vi "AIT 664 - Write FIFOs.vi"(0 "RT Data in":T2 {"End System Handle" format="%x"; "Label Transfer Config"."Block Data Refs"."Data Reference" format="%.0x"; "Status Config"."Hardware Out Dur Reference" format="%.0x"; "Status Config"."Hardware In Dur Reference" format="%.0x"; "Status Config"."Hardware Out Count Reference" format="%.0x"; "Status Config"."Hardware In Count Reference" format="%.0x"; "Status Config"."Error Data Reference" format="%.0x"; "Hardware Output Tx Channels"."Message Settings"."Transmit Channel Data Reference" format="%.0x"; "Hardware Output Tx Channels"."Message Settings"."Queue Transmit Channel" format="%.0x"; "Hardware Output Tx Channels"."Message Settings"."Driver Data"."Num Bits" min=1 max=32; "Hardware Output Tx Channels"."Message Settings"."Block Data Refs"."Data Reference" format="%.0x"; "Hardware Output Tx Channels"."Rx Com Udp Port"."Handle" format="%08x"; "Hardware Output Tx Channels"."Tx Com Udp Port"."Handle" format="%08x"; "Hardware Input Rx Channels"."Message Settings"."Transmit Channel Data Reference" format="%.0x"; "Hardware Input Rx Channels"."Message Settings"."Queue Transmit Channel" format="%.0x"; "Hardware Input Rx Channels"."Message Settings"."Driver Data"."Num Bits" min=1 max=32; "Hardware Input Rx Channels"."Message Settings"."Block Data Refs"."Data Reference" format="%.0x"; "Hardware Input Rx Channels"."Rx Com Udp Port"."Handle" format="%08x"; "Hardware Input Rx Channels"."Tx Com Udp Port"."Handle" format="%08x"}, 2 "Mode":T1, 5 "Channel Index":i32, 11 "error in (no error)":errorcluster) -> (4 "RT Data out":T2 {"End System Handle" format="%x"; "Label Transfer Config"."Block Data Refs"."Data Reference" format="%.0x"; "Status Config"."Hardware Out Dur Reference" format="%.0x"; "Status Config"."Hardware In Dur Reference" format="%.0x"; "Status Config"."Hardware Out Count Reference" format="%.0x"; "Status Config"."Hardware In Count Reference" format="%.0x"; "Status Config"."Error Data Reference" format="%.0x"; "Hardware Output Tx Channels"."Message Settings"."Transmit Channel Data Reference" format="%.0x"; "Hardware Output Tx Channels"."Message Settings"."Queue Transmit Channel" format="%.0x"; "Hardware Output Tx Channels"."Message Settings"."Driver Data"."Num Bits" min=1 max=32; "Hardware Output Tx Channels"."Message Settings"."Block Data Refs"."Data Reference" format="%.0x"; "Hardware Output Tx Channels"."Rx Com Udp Port"."Handle" format="%08x"; "Hardware Output Tx Channels"."Tx Com Udp Port"."Handle" format="%08x"; "Hardware Input Rx Channels"."Message Settings"."Transmit Channel Data Reference" format="%.0x"; "Hardware Input Rx Channels"."Message Settings"."Queue Transmit Channel" format="%.0x"; "Hardware Input Rx Channels"."Message Settings"."Driver Data"."Num Bits" min=1 max=32; "Hardware Input Rx Channels"."Message Settings"."Block Data Refs"."Data Reference" format="%.0x"; "Hardware Input Rx Channels"."Rx Com Udp Port"."Handle" format="%08x"; "Hardware Input Rx Channels"."Tx Com Udp Port"."Handle" format="%08x"}, 15 "error out":errorcluster)   [LabVIEW 2013, in "AIT 664 Custom Device.lvlib"]
doc: "Move data from the buffers to the FIFOs.\n\nInline Write - Data from Veristand to Hardware Out Buffer to the Hardware Out FIFO\nAsync HWIn - Data from device to Hardware In Buffer to the Hardware In FIFO"
uses:
  AIT 664 Custom Device.lvlib
  RT Controls/AIT 664  - RT Data.ctl
  RT Controls/AIT 664 - RT Hardware Channel.ctl
  RT Controls/AIT 664 - RT Message Settings.ctl
  <vilib>/NI Veristand/Custom Device API/Block Data Reference.ctl
  <vilib>/NI Veristand/Custom Device API/Data Reference.ctl
  RT Controls/AIT 664 - Driver Data.ctl
  Controls and Global/Start Bit.ctl
  Controls and Global/Number of Bits.ctl
  <vilib>/NI Veristand/Custom Device API/Custom Device Item Ref.ctl
  <userlib>/ARINC 664/AIT 664 Controls/General/Message Port.ctl
  <userlib>/ARINC 664/AIT 664 Controls/General/Direction.ctl
  <userlib>/ARINC 664/AIT 664 Controls/General/Message Port Type.ctl
  System Explorer/Controls/664 - Sampling Type.ctl
  RT Controls/Status Channels Config.ctl
  RT Controls/FIFO.ctl
  RT Controls/Label Transfer Config.ctl
  RT Controls/ReadWrite Selector.ctl
  <vilib>/NI Veristand/Custom Device API/Custom Device API.lvlib
  <userlib>/ARINC 664/AIT 664 API.lvlib
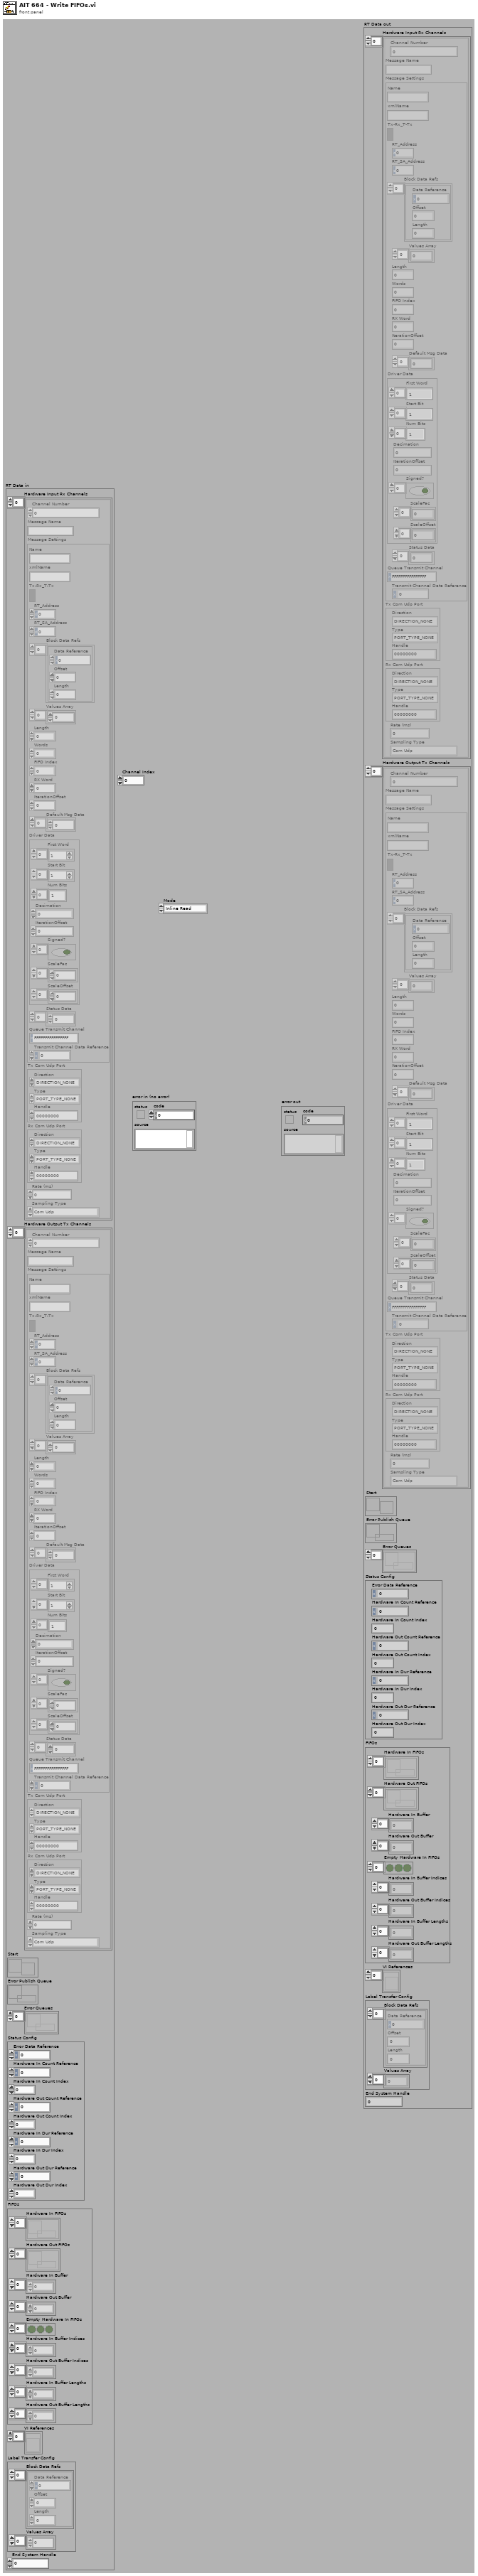
[diagram p1: front panel]
types:
  T1 = typedef "AIT 664 Custom Device.lvlib/ReadWrite Selector.ctl" = enum16{"Inline Read", "Inline Write", "Async HWIn", "Async HWOut"}
  T2 = typedef "AIT 664 Custom Device.lvlib/AIT 664  - RT Data.ctl" = cluster{"Hardware Input Rx Channels":T3[], "Hardware Output Tx Channels":T3[], "Start":refnum<notifier>, "Error Publish Queue":refnum<queue>, "Error Queues":refnum<queue>[], "Status Config":T15, "FIFOs":T16, "VI References":refnum<vi>[], "Label Transfer Config":T17, "End System Handle ":u64}
  T3 = typedef "AIT 664 Custom Device.lvlib/AIT 664 - RT Hardware Channel.ctl" = cluster{"Channel Number":u16, "Message Name":string, "Message Settings":T4, "Tx Com Udp Port":T11, "Rx Com Udp Port":T11, "Rate (ms)":u32, "Sampling Type":T14}
  T4 = typedef "AIT 664 Custom Device.lvlib/AIT 664 - RT Message Settings.ctl" = cluster{"Name":string, "xmlName":string, "Tx-Rx_T-Tx":bool, "RT_Address":u8, "RT_SA_Address":u8, "Block Data Refs":T5[], "Values Array":dbl[], "Length":i32, "Words":i32, "FIFO Index":i32, "RX Word":u32, "IterationOffset":i32, "Default Msg Data":u8[], "Driver Data":T7, "Status Data":u32[], "Queue Transmit Channel":T10, "Transmit Channel Data Reference":T6}
  T5 = typedef "Custom Device API.lvlib/Block Data Reference.ctl" = cluster{"Data Reference":T6, "Offset":i32, "Length":i32}
  T6 = typedef "Custom Device API.lvlib/Data Reference.ctl" = i32
  T7 = typedef "AIT 664 Custom Device.lvlib/AIT 664 - Driver Data.ctl" = cluster{"First Word":T8[], "Start Bit":T8[], "Num Bits":T9[], "Decimation":i32, "IterationOffset":i32, "Signed?":bool[], "ScaleFac":dbl[], "ScaleOffset":dbl[]}
  T8 = typedef "AIT 664 Custom Device.lvlib/Start Bit.ctl" = i32
  T9 = typedef "AIT 664 Custom Device.lvlib/Number of Bits.ctl" = i32
  T10 = typedef "Custom Device API.lvlib/Custom Device Item Ref.ctl" = u64
  T11 = typedef "AIT 664 API.lvlib/Message Port.ctl" = cluster{"Direction":T12, "Type":T13, "Handle":u64}
  T12 = typedef "AIT 664 API.lvlib/Direction.ctl" = enum16{"DIRECTION_NONE", "DIRECTION_TX", "DIRECTION_RX"}
  T13 = typedef "AIT 664 API.lvlib/Message Port Type.ctl" = enum16{"PORT_TYPE_NONE", "COM_UDP", "SAP_UDP", "SAP_IP", "SAP_MAC", "COTS_MAC", "COTS_MAC_RAW"}
  T14 = typedef "AIT 664 Custom Device.lvlib/664 - Sampling Type.ctl" = enum16{"Com Udp", "Com Udp Queuing", "Sap Udp", "Sap Ip", "Sap Mac", "Unknown"}
  T15 = typedef "AIT 664 Custom Device.lvlib/Status Channels Config.ctl" = cluster{"Error Data Reference":T6, "Hardware In Count Reference":T6, "Hardware In Count Index":i32, "Hardware Out Count Reference":T6, "Hardware Out Count Index":i32, "Hardware In Dur Reference":T6, "Hardware In Dur Index":i32, "Hardware Out Dur Reference":T6, "Hardware Out Dur Index":i32}
  T16 = typedef "AIT 664 Custom Device.lvlib/FIFO.ctl" = cluster{"Hardware In FIFOs":refnum<k33>[], "Hardware Out FIFOs":refnum<k33>[], "Hardware In Buffer":dbl[], "Hardware Out Buffer":dbl[], "Empty Hardware In FIFOs":bool[], "Hardware In Buffer Indices":i32[], "Hardware Out Buffer Indices":i32[], "Hardware In Buffer Lengths":i32[], "Hardware Out Buffer Lengths":i32[]}
  T17 = typedef "AIT 664 Custom Device.lvlib/Label Transfer Config.ctl" = cluster{"Block Data Refs":T5[], "Values Array":dbl[]}
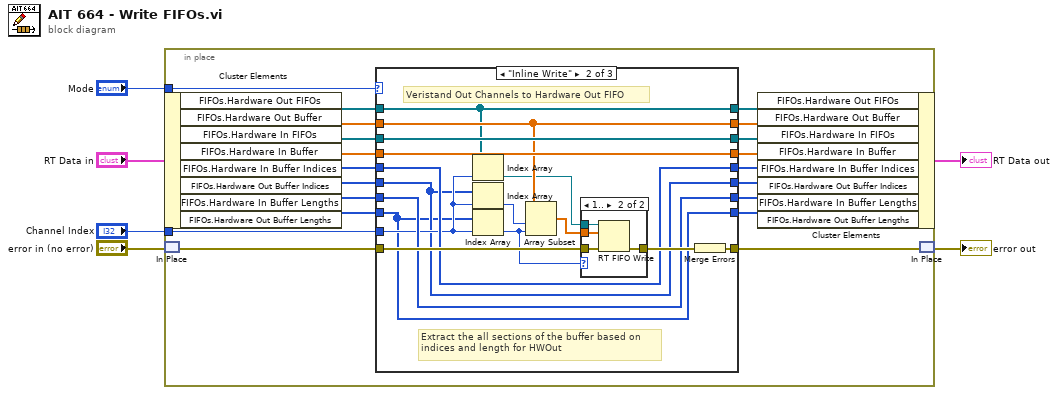
[diagram p0: block diagram]
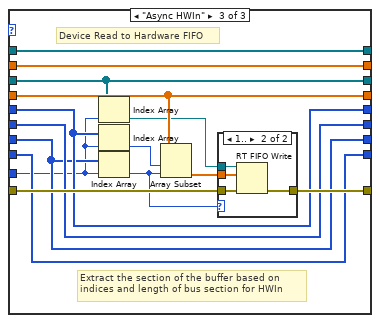
[diagram p4: hidden frame]
diagram:
  n1 = in-place {
    in-place-border: "Mode" -> [w20]
    in-place-border: "Channel Index" -> [w7]
    n2 = in-place-cluster #1("RT Data in") -> ("FIFOs.Hardware Out FIFOs"=w19:refnum<k33>[], "FIFOs.Hardware Out Buffer"=w18:dbl[], "FIFOs.Hardware In FIFOs"=w26:refnum<k33>[], "FIFOs.Hardware In Buffer"=w25:dbl[], "FIFOs.Hardware In Buffer Indices"=w15:i32[], "FIFOs.Hardware Out Buffer Indices"=w14:i32[], "FIFOs.Hardware In Buffer Lengths"=w13:i32[], "FIFOs.Hardware Out Buffer Lengths"=w12:i32[])
    n3 = in-place-match #2("error in (no error)") -> (w22:errorcluster)
    n4 = case shown="\"Inline Write\"" w20 {
      tunnel: w26 -> [w34 w49 w60]
      tunnel: w25 -> [w35 w50 w65]
      tunnel: [w35 w50 w65] -> w24
      tunnel: [w34 w49 w60] -> w23
      tunnel: w22 -> [w33 w51 w69]
      tunnel: [w33 w46 w68] -> w21
      tunnel: w19 -> [w31 w45 w71]
      tunnel: w18 -> [w32 w47 w70]
      tunnel: [w31 w45 w71] -> w17
      tunnel: [w32 w47 w70] -> w16
      tunnel: [w30 w43 w63] -> w11
      tunnel: w15 -> [w30 w43 w63]
      tunnel: [w29 w37 w66] -> w10
      tunnel: w14 -> [w29 w37 w66]
      tunnel: [w28 w42 w62] -> w9
      tunnel: w13 -> [w28 w42 w62]
      tunnel: [w27 w36 w67] -> w8
      tunnel: w12 -> [w27 w36 w67]
      tunnel: w7 -> [_ w41 w59]
      frame Default {
      }
      frame "Inline Write" {
        # "Veristand Out Channels to Hardware Out FIFO"
        # "Extract the all sections of the buffer based on \nindices and length for HWOut"
        n5 = Index Array(array=w45, index=w41) -> (element=w44:refnum<k33>)
        n6 = Index Array(array=w37, index=w41) -> (element=w40:i32)
        n7 = Index Array(array=w36, index=w41) -> (element=w38:i32)
        n8 = Array Subset(array=w47, index=w40, length=w38) -> (w39:dbl[])
        n9 = case shown="1.." w38 {
          tunnel: w51 -> [w52 w56]
          tunnel: [w52 w55] -> w48
          tunnel: w44 -> [_ w54]
          tunnel: w39 -> [_ w53]
          frame 0, Default {
          }
          frame 1.. {
            n10 = RT FIFO Write(0:w54, 1:w53, 3:w56) -> (11:w55:errorcluster)  [unwired: 2 in, 3 out]
          }
        }
        n11 = Merge Errors(w48) -> (w46:errorcluster)
      }
      frame "Async HWIn" {
        # "Device Read to Hardware FIFO"
        # "Extract the section of the buffer based on \nindices and length of bus section for HWIn"
        n12 = Index Array(array=w60, index=w59) -> (element=w58:refnum<k33>)
        n13 = Index Array(array=w63, index=w59) -> (element=w61:i32)
        n14 = Index Array(array=w62, index=w59) -> (element=w57:i32)
        n15 = Array Subset(array=w65, index=w61, length=w57) -> (w64:dbl[])
        n16 = case shown="1.." w57 {
          tunnel: w69 -> [w72 w76]
          tunnel: [w72 w75] -> w68
          tunnel: w64 -> [_ w74]
          tunnel: w58 -> [_ w73]
          frame 0, Default {
          }
          frame 1.. {
            n17 = RT FIFO Write(0:w73, 1:w74, 3:w76) -> (11:w75:errorcluster)  [unwired: 2 in, 3 out]
          }
        }
      }
    }
    n18 = in-place-cluster #1("FIFOs.Hardware Out FIFOs"=w17, "FIFOs.Hardware Out Buffer"=w16, "FIFOs.Hardware In FIFOs"=w23, "FIFOs.Hardware In Buffer"=w24, "FIFOs.Hardware In Buffer Indices"=w11, "FIFOs.Hardware Out Buffer Indices"=w10, "FIFOs.Hardware In Buffer Lengths"=w9, "FIFOs.Hardware Out Buffer Lengths"=w8) -> (→"RT Data out":T2)
    n19 = in-place-match #2(w21) -> (→"error out":errorcluster)
  }
